vi "Test_Billede.vi"() -> ()   [LabVIEW 2018]
panel:
  in  "stop":bool
  out "Image 4":T1(plugin-control)
  out "Image 3":T1(plugin-control)
  out "Image 2":T1(plugin-control)
  out "Image":T1(plugin-control)
  out "Image Out":T1(plugin-control)
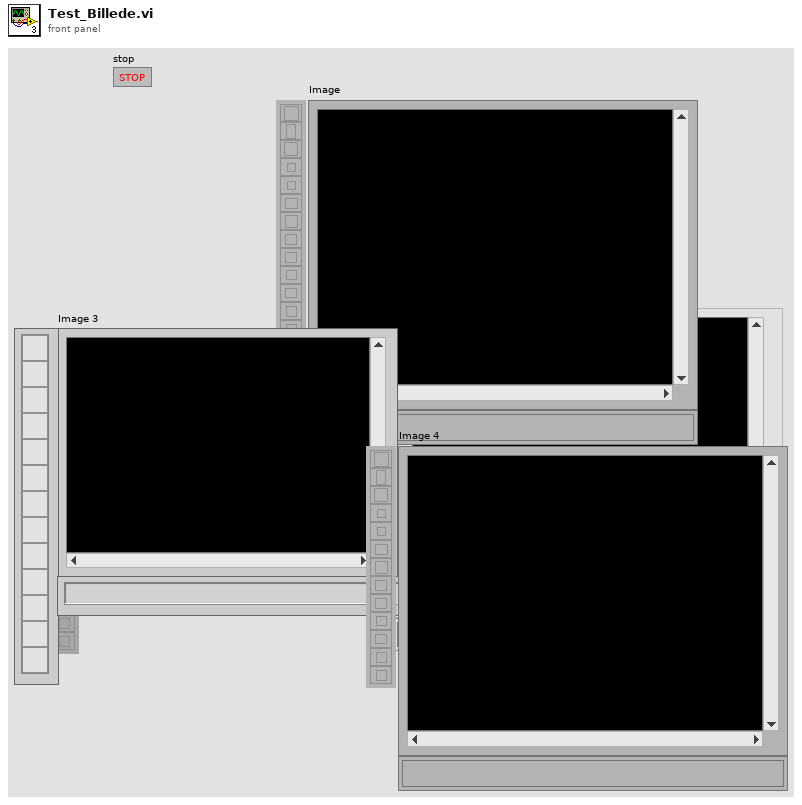
[diagram p1: front panel]
types:
  T1 = typedef "IMAQ Image.ctl" = refnum<image>
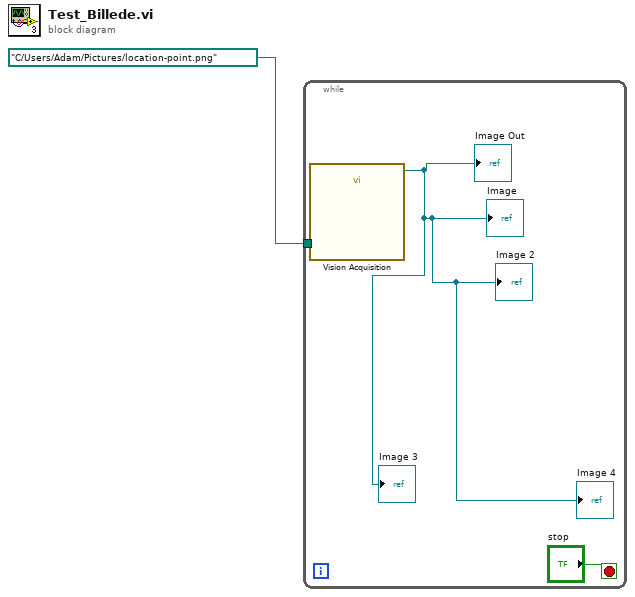
[diagram p0: block diagram]
diagram:
  n1 = while {
    tunnel: path "C:/Users/Adam/Pictures/location-point.png" ("Image Path") -> [w4]
    stop <- "stop" stop-if-true
    n2 = call "Vision Acquisition"("Image Path"=w4) -> ("Image Out"=→"Image Out" →"Image" →"Image 2" →"Image 3" →"Image 4":T1)  [unwired: 25 in, 1 out]
  }
